vi "Calibration.vi"(0 "FileHandle in":refnum<k24>, 1 "PosList":refnum<vi>, 2 "ANDORExposure":sgl, 3 "ValveRing":T8(ring), 4 "ProgramSingleMultiring":u16, 5 "error in (no error)":errorcluster, 6 "Clust Refnum":refnum<vi>, 7 "ValveReagent":T8(ring), 8 "Dilution Step":i32, 9 "Calib Feed Cycles":u8, 10 "LINX Resource":T1, 11 "Calib Mix Cycles":u16, 12 "Image Number":i32, 13 "TANGO":i32) -> (14 "FileHandle out":refnum<k24>, 15 "LINX Resource out":T1, 16 "Image":T7, 17 "Remaining Time":dbl, 19 "error out":errorcluster)   [LabVIEW 2018]
uses:
  C:/Users/Familie/Documents/LabviewIX81/lib/tiff/LVTiffWriter/BitMiracle.LibTiff.NET.dll
  tiff/LVTiffWriter/BitMiracle.LibTiff.NET.dll
  <vilib>/vision/Image Controls.llb/IMAQ Image.ctl
  <vilib>/MakerHub/LINX/Private/Type Defs/LINX Ref.ctl
  <vilib>/MakerHub/LINX/Private/Type Defs/Platform.ctl
  <vilib>/MakerHub/LINX/Private/Type Defs/Interface.ctl
  <vilib>/MakerHub/LINX/Private/Device/Type Defs/LINX Device Config.ctl
  <vilib>/MakerHub/LINX/Private/Device/Type Defs/TCP Config.ctl
  <vilib>/MakerHub/LINX/Private/Device/Type Defs/Channels.ctl
  Arduino/VIs/Arduino.lvlib
  Calibration.lvlib
  <vilib>/MakerHub/LINX/LMH-LINX.lvlib
  <vilib>/MakerHub/LINX/Private/Device/Device.lvlib
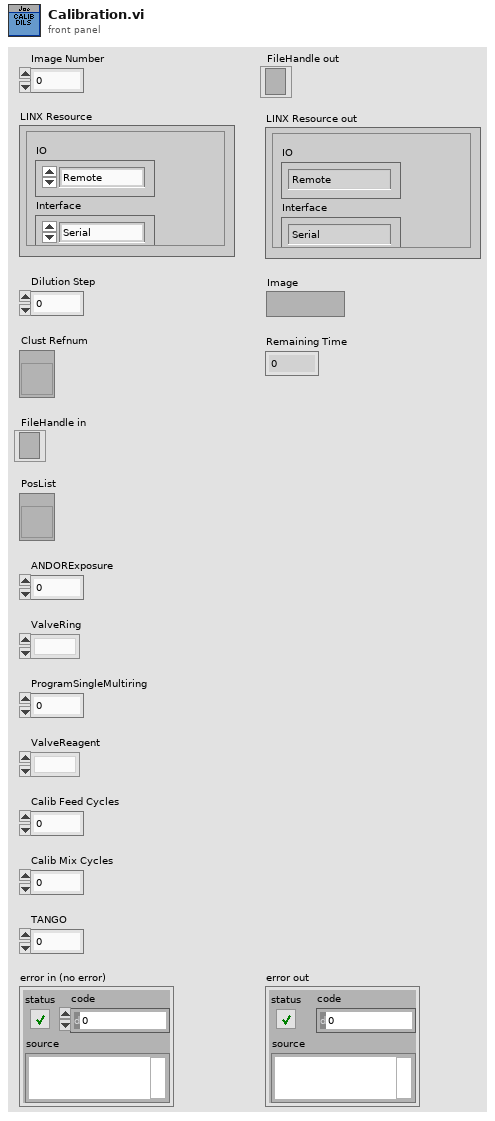
[diagram p1: front panel]
types:
  T1 = typedef "LMH-LINX.lvlib/LINX Ref.ctl" = cluster{"IO":T2, "Interface":T3, "LINX Device Config":T4}
  T2 = typedef "LMH-LINX.lvlib/Platform.ctl" = enum16{"Remote", "Local"}
  T3 = typedef "LMH-LINX.lvlib/Interface.ctl" = enum16{"Serial", "TCP"}
  T4 = typedef "LMH-LINX.lvlib/Device.lvlib/LINX Device Config.ctl" = cluster{"Interface":T3, "COM Port":refnum<visa-resource-name>, "TCP Configuration":T5, "Device Family":u8, "Device ID":u8, "Device Name":string, "TCP Ref":refnum<k5>, "Channels":T6}
  T5 = typedef "LMH-LINX.lvlib/Device.lvlib/TCP Config.ctl" = cluster{"IP Address":string, "Port":u16}
  T6 = typedef "LMH-LINX.lvlib/Channels.ctl" = cluster{"DI":u8[], "DO":u8[], "AI":u8[], "AO":u8[], "PWM":u8[], "QE":u8[], "UART":u8[], "I2C 2":u8[], "SPI":u8[], "CAN":u8[], "Servo":u8[], "AI Ref (V)":dbl, "AI Resolution (Bits)":u8, "AO Ref (V)":dbl, "AO Resolution (Bits)":u8}
  T7 = typedef "IMAQ Image.ctl" = refnum<image>
  T8 = enum8{"", "1", "2", "3", "4", "5", "6", "7", "8"}
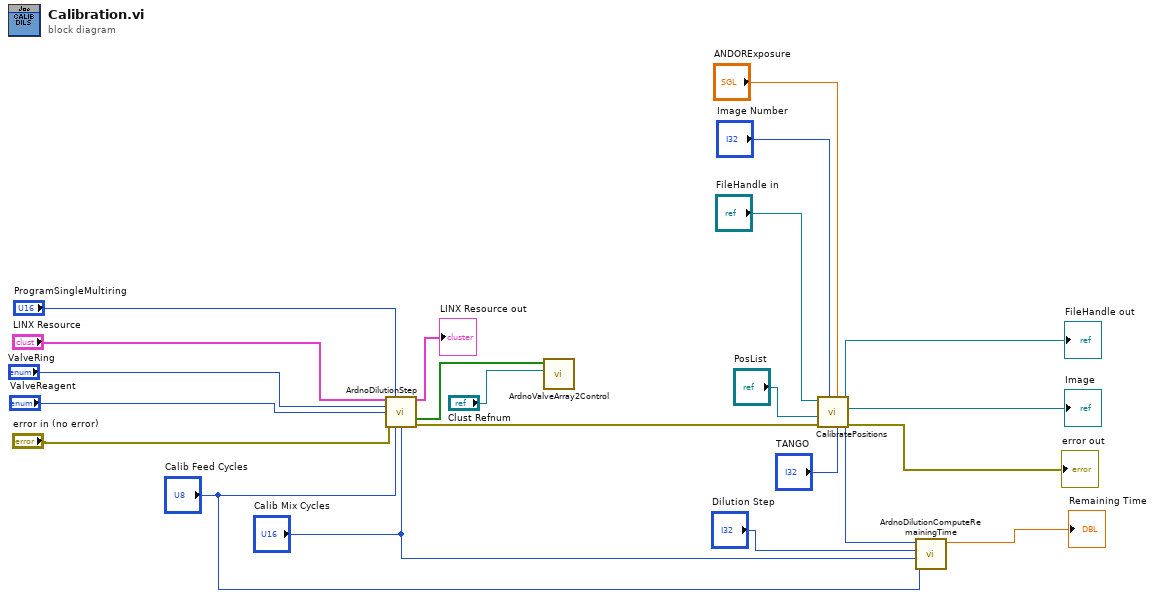
[diagram p0: block diagram]
diagram:
  n1 = call "ArdnoDilutionStep.vi"("LINX Resource"="LINX Resource", "Single / Multiring?"="ProgramSingleMultiring", "Ring"="ValveRing", "Channel"="ValveReagent", "error in (no error)"="error in (no error)", "Feed Cycles"="Calib Feed Cycles", "Mix Cycles"="Calib Mix Cycles") -> ("LINX Resource out"=→"LINX Resource out":T1, "ValveStates"=w19:bool[], "error out"=w6:errorcluster)  [unwired: 6 in]
  n2 = call "ArdnoValveArray2Control.vi"("Cluster in"="Clust Refnum", "ValveStates"=w19) -> ()  [unwired: 10 in]
  n3 = call "CalibratePositions.vi"("TANGO"="TANGO", "ANDORExposure"="ANDORExposure", "CalibStep"="Image Number", "error in (no error)"=w6, "PosList"="PosList", ".NET Refnum in"="FileHandle in") -> ("error out"=→"error out":errorcluster, "Elaspsed [ms]"=w16:u32, "Image"=→"Image":T7, ".NET Refnum out"=→"FileHandle out":refnum<k24>)  [unwired: 2 in]
  n4 = call "ArdnoDilutionComputeRemainingTime.vi"("Calib Feed Cycles"="Calib Feed Cycles", "Calib Mix Cycles"="Calib Mix Cycles", "Dilution Step"="Dilution Step", "Acquisition Time"=w16) -> ("Remaining Time"=→"Remaining Time":dbl)  [unwired: 7 in]
